vi "Timer.vi"(8 "error in (no error)":errorcluster, 11 "Enum":T1(ring)) -> (0 "error out":errorcluster, 3 "Numeric":sgl)   [LabVIEW 2019]
doc: "Simple timer VI with \"reset\" and \"get time\" functions."
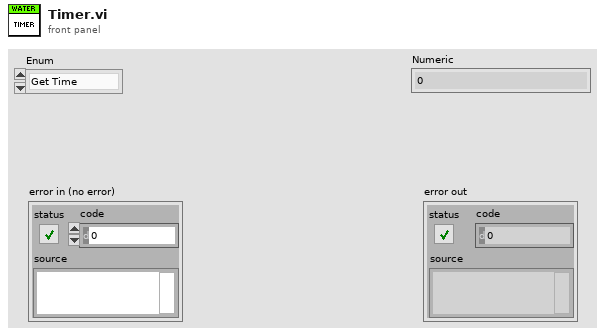
[diagram p1: front panel]
types:
  T1 = enum16{"Get Time", "Reset Time", "Pause", "Resume"}
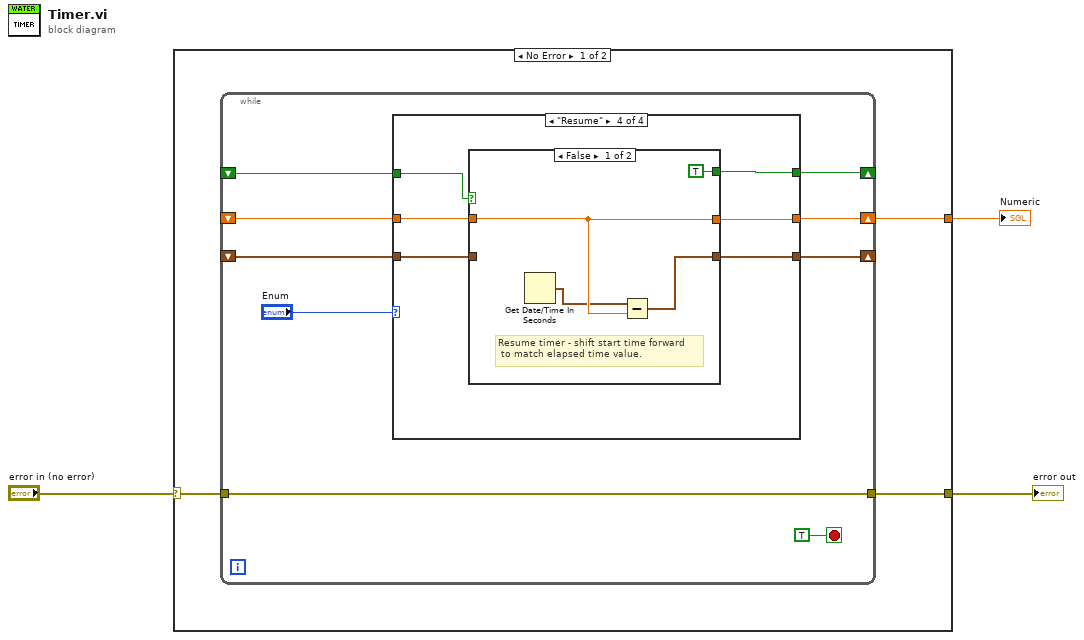
[diagram p0: block diagram]
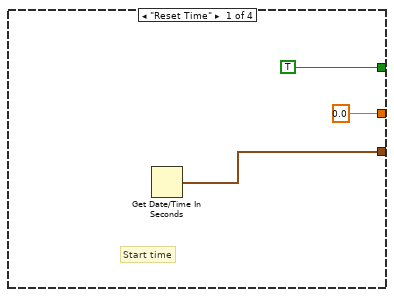
[diagram p2: hidden frame]
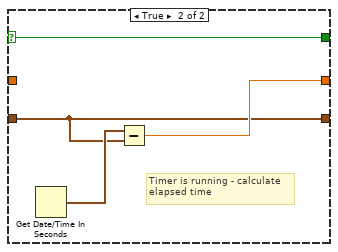
[diagram p4: hidden frame]
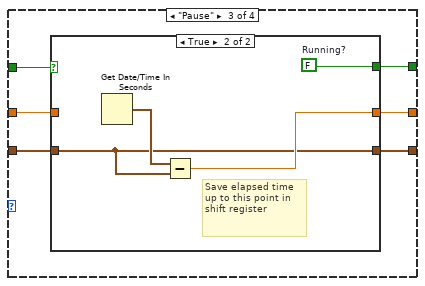
[diagram p5: hidden frame]
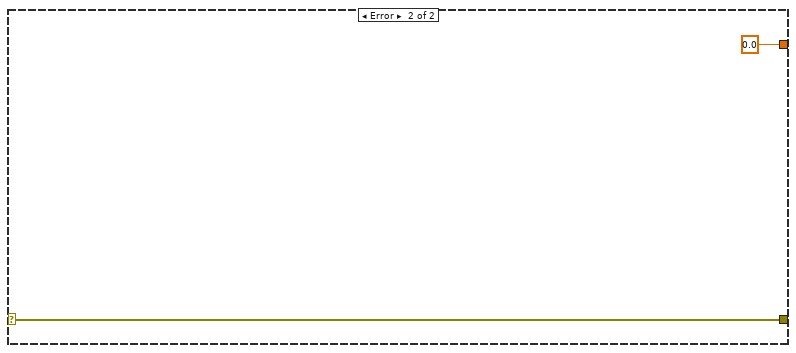
[diagram p8: hidden frame]
diagram:
  n1 = case shown="No Error" "error in (no error)" {
    selector: "error in (no error)" -> [w5 w59]
    tunnel: [w6 w59] -> w2
    tunnel: [w4 0.0] -> w1
    frame No Error {
      n2 = while {
        shift-right: [w13] -> w4
        shift-left: _ -> [w9]
        shift-right: [w12] -> _
        shift-left: _ -> [w15]
        tunnel: [w10] -> w6
        tunnel: w5 -> [w10]
        shift-right: [w8] -> _
        shift-left: _ -> [w7]
        stop <- TRUE stop-if-true
        n3 = case shown="\"Resume\"" "Enum" {
          tunnel: [w18 w19 w33 w49] -> w12
          tunnel: w15 -> [_ w23 w36 w48]
          tunnel: [sgl 0.0 ("Numeric") w24 w37 w47] -> w13
          tunnel: w9 -> [_ w21 w32 w50]
          tunnel: [TRUE ("Running?") w20 w35 w45] -> w8
          tunnel: w7 -> [_ w22 w34 w46]
          frame "Reset Time" {
            # "Start time"
            n4 = Get Date/Time In Seconds() -> (seconds since 1Jan1904=w18:timestamp)
          }
          frame "Get Time", Default {
            n5 = case shown="False" w22 {
              selector: w22 -> [w26 w29]
              tunnel: [w27 w31] -> w24
              tunnel: w23 -> [w25 w28]
              tunnel: w21 -> [w27 _]
              tunnel: [w26 w29] -> w20
              tunnel: [w25 w28] -> w19
              frame False {
                # "Timer is not running pass\nlast value of elapsed time"
              }
              frame True {
                # "Timer is running - calculate\nelapsed time"
                n6 = Get Date/Time In Seconds() -> (seconds since 1Jan1904=w30:timestamp)
                n7 = Subtract(x=w30, y=w28) -> (x-y=w31:dbl)
              }
            }
          }
          frame "Pause" {
            n8 = case shown="True" w34 {
              selector: w34 -> [w38 _]
              tunnel: [w39 w43] -> w37
              tunnel: w36 -> [w40 w41]
              tunnel: [w38 w42] -> w35
              tunnel: [w40 w41] -> w33
              tunnel: w32 -> [w39 _]
              frame False {
                # "Already paused, do nothing"
              }
              frame True {
                w42 = FALSE  # Running?
                # "Save elapsed time up to this point in shift register"
                n9 = Get Date/Time In Seconds() -> (seconds since 1Jan1904=w44:timestamp)
                n10 = Subtract(x=w44, y=w41) -> (x-y=w43:dbl)
              }
            }
          }
          frame "Resume" {
            n11 = case shown="False" w46 {
              selector: w46 -> [_ w55]
              tunnel: w50 -> [w53 w57]
              tunnel: [w54 w56] -> w49
              tunnel: w48 -> [_ w56]
              tunnel: [w53 w57] -> w47
              tunnel: [TRUE w55] -> w45
              frame False {
                # "Resume timer - shift start time forward\n to match elapsed time value."
                n12 = Get Date/Time In Seconds() -> (seconds since 1Jan1904=w51:timestamp)
                n13 = Subtract(x=w51, y=w53) -> (x-y=w54:timestamp)
              }
              frame True {
                # "Already running, do nothing"
              }
            }
          }
        }
      }
    }
    frame Error {
    }
  }
  "error out" <- w2
  "Numeric" <- w1
